vi "day 12 task 1 BFS.vi"() -> ()   [LabVIEW 2019]
panel:
  out "Numeric":i32
  out "size(s)":i32
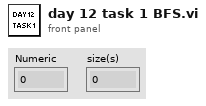
[diagram p1: front panel]
types:
  T1 = cluster{"current location":cluster{"x":i32, "y":i32}, "goal location":cluster{"x":i32, "y":i32}, "visited":bool[][], "heightmap":u8[][], "lettermap":string[][], "visited":cluster{"x":i32, "y":i32}[], "stack":cluster{"x":i32, "y":i32}[], "Joined parent of visited":u64[]}
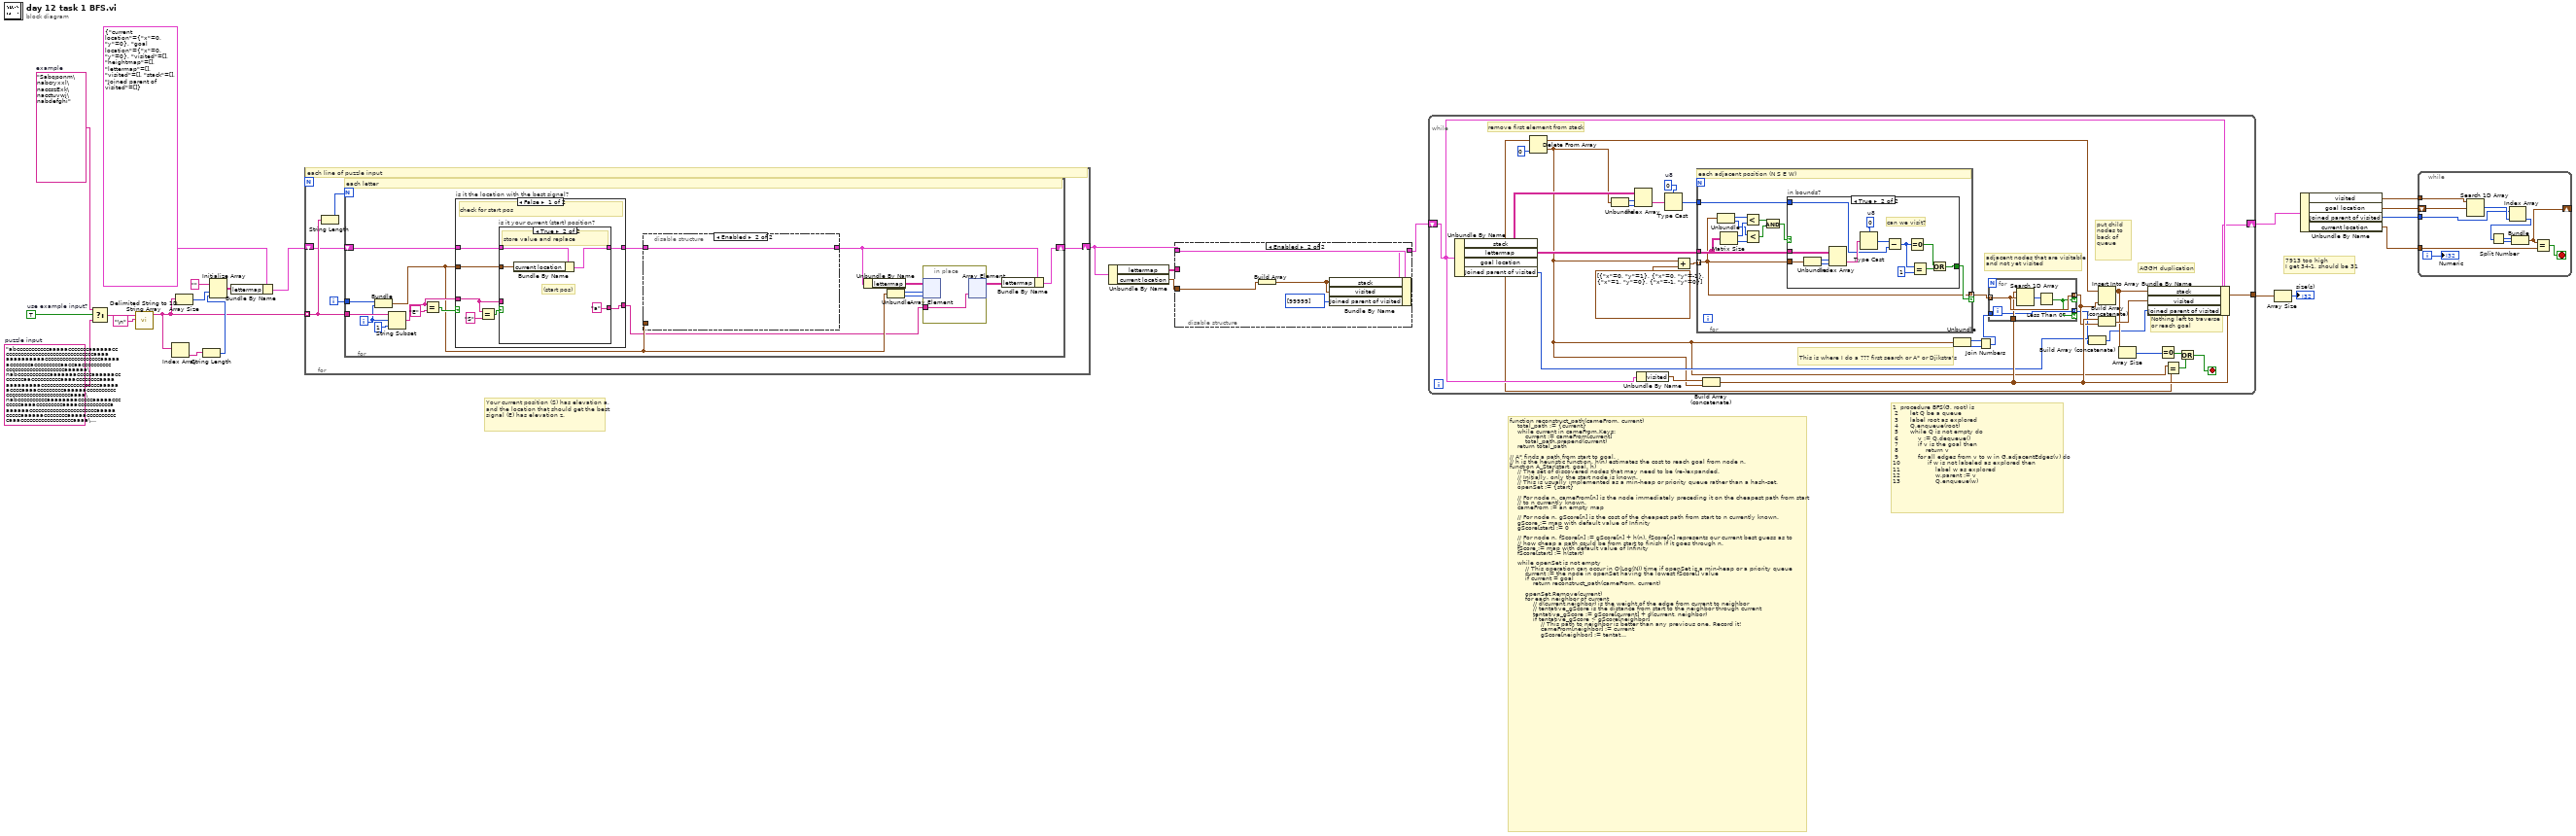
[diagram p0: block diagram]
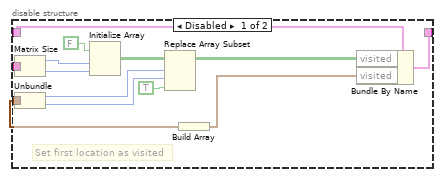
[diagram p3: hidden frame]
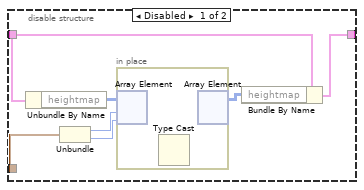
[diagram p4: hidden frame]
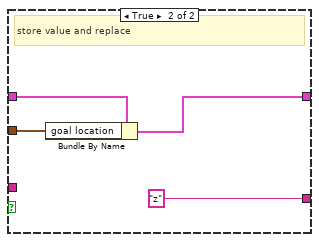
[diagram p6: hidden frame]
diagram:
  w22 = "Sabqponm\nabcryxxl\naccszExk\nacctuvwj\nabdefghi"  # example
  w23 = TRUE  # use example input?
  w24 = "abcccccccccccaaaaacccccccaaaaaaccccccccccccccccccccccccccccccccaaaaaaaaaaaaaacccccccccccccccccccaaaaaacccccccacccccccccaaccaaccccccccccccccccccccccccccccccaaaaaa\nabcccccccccccaaaaaaacccccaaaaaaccccccccaaccccccccccaaaaccccccccaaaaaaaaaaaaaccccccccccccccccccccaaaaaaccccaaaacccccccccaaaaaaccccccccccccccccccccccccccccccccaaaa\nabccccccccccaaaaaaaacccccaaaaaccccccccaaaacccccccccaaaacccccccccccaaaaaaacccccccccccccccccccccccaaaaacccccaaaaaaccccccccaaaaacccccccccccaaaccccccccccccccccccaaaa\nabccccccccccaaaaaaaaccccccaaaaacccccccaaaacccccccccaaaacccccaaaccccaaaaaaccccccccccccccccccccccccaaaaacccccaaaaacc..."  # puzzle input
  # "7913 too high\nI get 34-1, should be 31"
  # "1  procedure BFS(G, root) is\n 2      let Q be a queue\n 3      label root as explored\n 4      Q.enqueue(root)\n 5      while Q is not empty do\n 6          v := Q.dequeue()\n 7          if v is the goal then\n 8              return v\n 9          for all edges from v to w in G.adjacentEdges(v) do\n10              if w is not labeled as explored then\n11                  label w as explored\n12                  w.parent := v\n13                  Q.enqueue(w)"
  # "function reconstruct_path(cameFrom, current)\n    total_path := {current}\n    while current in cameFrom.Keys:\n        current := cameFrom[current]\n        total_path.prepend(current)\n    return total_path\n\n// A* finds a path from start to goal.\n// h is the heuristic function. h(n) estimates the cost to reach goal from node n.\nfunction A_Star(start, goal, h)\n    // The set of discovered nodes that may need to be (re-)expanded.\n    // Initially, only the start node is known.\n    // This is usually implemented as a min-heap or priority queue rather than a hash-set.\n    openSet := {start}\n\n    // For node n, cameFrom[n] is the node immediately preceding it on the cheapest path from start\n    // to n currently known.\n    cameFrom := an empty map\n\n    // For node n, gScore[n] is the cost of the cheapest path from start to n currently known.\n    gScore := map with default value of Infinity\n    gScore[start] := 0\n\n    // For node n, fScore[n] := gScore[n] + h(n). fScore[n] represents our current best guess as to\n    // how cheap a path could be from start to finish if it goes through n.\n    fScore := map with default value of Infinity\n    fScore[start] := h(start)\n\n    while openSet is not empty\n        // This operation can occur in O(Log(N)) time if openSet is a min-heap or a priority queue\n        current := the node in openSet having the lowest fScore[] value\n        if current = goal\n            return reconstruct_path(cameFrom, current)\n\n        openSet.Remove(current)\n        for each neighbor of current\n            // d(current,neighbor) is the weight of the edge from current to neighbor\n            // tentative_gScore is the distance from start to the neighbor through current\n            tentative_gScore := gScore[current] + d(current, neighbor)\n            if tentative_gScore < gScore[neighbor]\n                // This path to neighbor is better than any previous one. Record it!\n                cameFrom[neighbor] := current\n                gScore[neighbor] := tentative_gScore\n                fScore[neighbor] := tentative_gScore + h(neighbor)\n                if neighbor not in openSet\n                    openSet.add(neighbor)\n\n    // Open set is empty but goal was never reached\n    return failure"
  # "Your current position (S) has elevation a, and the location that should get the best signal (E) has elevation z."
  n1 = Select(t=w22, s=w23, f=w24) -> (s? t:f=w21:string)
  n2 = call <vilib>:"Delimited String to 1D String Array.vi"("delimiter"="\n" ("regular expression"), "delimited string"=w21) -> ("string array"=w7:string[])  [unwired: 9 in]
  n3 = Index Array(array=w7) -> (element=w11:string)  [unwired: 1 in]
  n4 = Array Size(array=w7) -> (size(s)=w8:i32)
  n5 = String Length(string=w11) -> (length=w9:i32)
  n6 = Initialize Array("", w8, w9) -> (w6:string[][])
  n7 = Bundle By Name(cluster=T1 {"current location"={"x"=0, "y"=0}, "goal location"={"x"=0, "y"=0}, "visited"=[], "heightmap"=[], "lettermap"=[], "visited"=[], "stack"=[], "Joined parent of visited"=[]}, "lettermap"=w6) -> (w12:T1)
  n8 = for {
    tunnel: w7 -> [w28] mode=indexing
    shift-right: [w26] -> w18
    shift-left: w12 -> [w25]
    i -> [w27]
    # "each line of puzzle input"
    n9 = String Length(string=w28) -> (length=w29:i32)
    n10 = for {
      N: w29 -> [_]
      tunnel: w28 -> [w45]
      tunnel: w27 -> [w42]
      shift-right: [w30] -> w26
      shift-left: w25 -> [w40]
      i -> [w43]
      # "each letter"
      n11 = Bundle(w42, w43) -> (w38:cluster{i32, i32})  [unwired: 1 in]
      n12 = String Subset(string=w45, offset (0)=w43, length (rest)=1 ("length (rest)")) -> (substring=w39:string)
      n13 = Equal?(x=w39, y="E") -> (x = y?=w41:bool)
      n14 = case "is it the location with the best signal?" shown="False" w41 {
        tunnel: w40 -> [w60 w72]
        tunnel: w38 -> [w59 w71]
        tunnel: [w58 w70] -> w35
        tunnel: w39 -> [w56 _]
        tunnel: [w57 "z" ("y")] -> w33
        frame False {
          # "check for start pos"
          n15 = Equal?(x=w56, y="S") -> (x = y?=w61:bool)
          n16 = case "is it your current (start) position?" shown="True" w61 {
            tunnel: w60 -> [w64 w68]
            tunnel: w59 -> [_ w67]
            tunnel: [w64 w66] -> w58
            tunnel: [w63 "a" ("String")] -> w57
            tunnel: w56 -> [w63 _]
            frame False {
              # "just pass the letter through"
            }
            frame True {
              # "(start pos)"
              # "store value and replace"
              n17 = Bundle By Name(cluster=w68, "current location"=w67) -> (w66:T1)
            }
          }
        }
        frame True {
          # "store value and replace"
          n18 = Bundle By Name(cluster=w72, "goal location"=w71) -> (w70:T1)
        }
      }
      n19 = disable-structure shown="Enabled" {
        disable-tunnel: w38 -> [w50 _]
        disable-tunnel: w35 -> [w49 w54]
        disable-tunnel: [w48 w54] -> w31
        frame Disabled {
          n20 = Unbundle By Name(w49) -> ("heightmap"=w53:u8[][])
          n21 = Unbundle(w50) -> (w52:i32, w51:i32)
          n22 = in-place {
            n23 = in-place-array #1(w53, w52, w51) -> ()  [unwired: 1 out]
            n24 = Type Cast() -> ()  [unwired: 2 in, 1 out]
            n25 = in-place-array #1() -> (w47:u8[][])  [unwired: 1 in, 2 out]
          }
          n26 = Bundle By Name(cluster=w49, "heightmap"=w47) -> (w48:T1)
        }
        frame Enabled {
        }
      }
      n27 = Unbundle By Name(w31) -> ("lettermap"=w34:string[][])
      n28 = Unbundle(w38) -> (w37:i32, w36:i32)
      n29 = in-place {
        in-place-border: w33 -> [w55]
        n30 = in-place-array #2(w34, w37, w36) -> ()  [unwired: 1 out]
        n31 = in-place-array #2(w55) -> (w32:string[][])  [unwired: 2 out]
      }
      n32 = Bundle By Name(cluster=w31, "lettermap"=w32) -> (w30:T1)
    }
  }
  n33 = Unbundle By Name(w18) -> ("lettermap"=w19:string[][], "current location"=w16:cluster{"x":i32, "y":i32})
  n34 = disable-structure shown="Enabled" {
    disable-tunnel: w19 -> [w85 _]
    disable-tunnel: w18 -> [w77 w90]
    disable-tunnel: [w76 w88] -> w17
    disable-tunnel: w16 -> [w74 w89]
    frame Disabled {
      # "Set first location as visited"
      n35 = Matrix Size(0:w85) -> (1:w83:i32, 2:w82:i32)
      n36 = Unbundle(w74) -> ("x"=w80:i32, "y"=w79:i32)
      n37 = Initialize Array(FALSE, w83, w82) -> (w81:bool[][])
      n38 = Replace Array Subset(array=w81, new element=TRUE, index (row)=w80, index (col)=w79) -> (w75:bool[][])
      n39 = Build Array(w74) -> (w73:cluster{"x":i32, "y":i32}[])
      n40 = Bundle By Name(cluster=w77, "visited"=w75, "visited"=w73) -> (w76:T1)
    }
    frame Enabled {
      n41 = Build Array(w89) -> (w86:cluster{"x":i32, "y":i32}[])
      n42 = Bundle By Name(cluster=w90, "stack"=w86, "visited"=w86, "Joined parent of visited"=u64[] [99999]) -> (w88:T1)
    }
  }
  n43 = while {
    shift-right: [w104] -> w5
    shift-left: w17 -> [w106]
    tunnel: [w103] -> w15
    stop <- w107 stop-if-true
    w115 = u8 0  # u8
    # "AGGH duplication"
    # "put child nodes to back of queue"
    # "remove first element from stack"
    # "Nothing left to traverse \nor reach goal"
    # "adjacent nodes that are visitable\nand not yet visited"
    # "This is where I do a ??? first search or A* or Djikstra's"
    n44 = Unbundle By Name(w106) -> ("stack"=w112:cluster{"x":i32, "y":i32}[], "lettermap"=w117:string[][], "goal location"=w99:cluster{"x":i32, "y":i32}, "Joined parent of visited"=w94:u64[])
    n45 = Delete From Array(array=w112, index=0) -> (deleted portion=w92:cluster{"x":i32, "y":i32}, array with subset deleted=w110:cluster{"x":i32, "y":i32}[])  [unwired: 1 in]
    n46 = Unbundle(w92) -> ("x"=w119:i32, "y"=w118:i32)
    n47 = Index Array(array=w117, index (row)=w119, index (col)=w118) -> (element=w116:string)
    n48 = Unbundle By Name(w106) -> ("visited"=w105:cluster{"x":i32, "y":i32}[])
    n49 = Type Cast(type=w115, x=w116) -> (*(type *) &x=w114:u8)
    n50 = Add(x=w92, y=cluster{"x":i32, "y":i32}[] [{"x"=0, "y"=1}, {"x"=0, "y"=-1}, {"x"=1, "y"=0}, {"x"=-1, "y"=0}]) -> (x+y=w120:cluster{"x":i32, "y":i32}[])
    n51 = for {
      tunnel: w117 -> [w135]
      tunnel: w120 -> [w133] mode=indexing
      tunnel: w114 -> [w137]
      tunnel: [w133] -> w113 mode=indexing if=w136
      # "each adjacent position (N S E W)"
      n52 = Unbundle(w133) -> ("x"=w134:i32, "y"=w131:i32)
      n53 = Matrix Size(0:w135) -> (1:w132:i32, 2:w130:i32)
      n54 = Less?(x=w134, y=w132) -> (x < y?=w129:bool)
      n55 = Less?(x=w131, y=w130) -> (x < y?=w128:bool)
      n56 = And(x=w129, y=w128) -> (x .and. y?=w127:bool)
      n57 = case "in bounds?" shown="True" w127 {
        tunnel: w137 -> [_ w145]
        tunnel: [_ w140] -> w136
        tunnel: w135 -> [_ w139]
        tunnel: w133 -> [_ w138]
        frame False {
        }
        frame True {
          w148 = u8 0  # u8
          # "can we visit?"
          n58 = Unbundle(w138) -> ("x"=w150:i32, "y"=w149:i32)
          n59 = Index Array(array=w139, index (row)=w150, index (col)=w149) -> (element=w147:string)
          n60 = Type Cast(type=w148, x=w147) -> (*(type *) &x=w146:u8)
          n61 = Subtract(x=w146, y=w145) -> (x-y=w144:u8)
          n62 = Equal To 0?(x=w144) -> (x = 0?=w142:bool)
          n63 = Equal?(x=w144, y=u8 1) -> (x = y?=w141:bool)
          n64 = Or(x=w142, y=w141) -> (x .or. y?=w140:bool)
        }
      }
    }
    n65 = Build Array (concatenate)(w105, w92) -> (w103:cluster{"x":i32, "y":i32}[])
    n66 = Unbundle(w92) -> ("x"=w97:i32, "y"=w96:i32)
    n67 = Join Numbers(hi=w97, lo=w96) -> ((hi.lo)=w95:u64)
    n68 = for {
      tunnel: w113 -> [w125] mode=indexing
      tunnel: [w125] -> w102 mode=indexing if=w122
      tunnel: w103 -> [w124]
      tunnel: w95 -> [w123]
      tunnel: [w123] -> w91 mode=indexing if=w122
      n69 = Search 1D Array(1D array=w124, element=w125) -> (index of element=w126:i32)  [unwired: 1 in]
      n70 = Less Than 0?(x=w126) -> (x < 0?=w122:bool)
    }
    n71 = Build Array (concatenate)(w94, w91) -> (w93:u64[])
    n72 = Insert Into Array(array=w110, new element=w102) -> (w100:cluster{"x":i32, "y":i32}[])  [unwired: 1 in]
    n73 = Build Array (concatenate)(w103, w102) -> (w101:cluster{"x":i32, "y":i32}[])
    n74 = Array Size(array=w100) -> (size(s)=w108:i32)
    n75 = Bundle By Name(cluster=w106, "stack"=w100, "visited"=w101, "Joined parent of visited"=w93) -> (w104:T1)
    n76 = Equal To 0?(x=w108) -> (x = 0?=w109:bool)
    n77 = Equal?(x=w92, y=w99) -> (x = y?=w98:bool)
    n78 = Or(x=w109, y=w98) -> (x .or. y?=w107:bool)
  }
  n79 = Array Size(array=w15) -> (size(s)=→"size(s)":i32)
  n80 = Unbundle By Name(w5) -> ("visited"=w4:cluster{"x":i32, "y":i32}[], "goal location"=w3:cluster{"x":i32, "y":i32}, "Joined parent of visited"=w2:u64[], "current location"=w1:cluster{"x":i32, "y":i32})
  n81 = while {
    tunnel: w4 -> [w161]
    tunnel: w2 -> [w158]
    tunnel: w1 -> [w154]
    shift-right: [w151] -> _
    shift-left: w3 -> [w160]
    i -> [w152]
    stop <- w153 stop-if-true
    n82 = Search 1D Array(1D array=w161, element=w160) -> (index of element=w159:i32)  [unwired: 1 in]
    n83 = Index Array(array=w158, index=w159) -> (element=w155:u64)
    n84 = Split Number(x=w155) -> (hi(x)=w157:u32, lo(x)=w156:u32)
    n85 = Bundle(w157, w156) -> (w151:cluster{u32, u32})  [unwired: 1 in]
    n86 = Equal?(x=w151, y=w154) -> (x = y?=w153:bool)
    "Numeric" <- w152
  }
